vi "Graph_Scaler_rate.vi"(3 "Data in":dbl[](array[numeric])) -> (1 "Data out":T1)   [LabVIEW 2014]
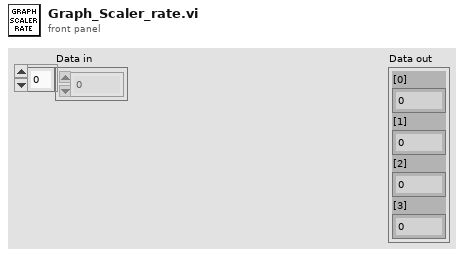
[diagram p1: front panel]
types:
  T1 = cluster{"[0]":dbl, "[1]":dbl, "[2]":dbl, "[3]":dbl}
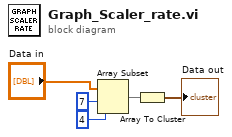
[diagram p0: block diagram]
diagram:
  n1 = Array Subset(array="Data in", index=7, length=4) -> (w1:dbl[])
  n2 = Array To Cluster(array=w1) -> (cluster=→"Data out":T1)
